vi "VI Tree.vi"   [LabVIEW 2012, in "Temptronic TP04300.lvlib"]
doc: "This is the instrument driver for the Temptronic 4300. The VI Tree displays all the user-callable VIs of the instrument driver in an organized table."
uses:
  <instrlib>/Temptronic TP04300/Temptronic TP04300.lvlib
panel:
  # "© 2007 Temptronic Corporation.  ALL RIGHTS RESERVED."
  # "SEE DIAGRAM\nFOR VI TREE."
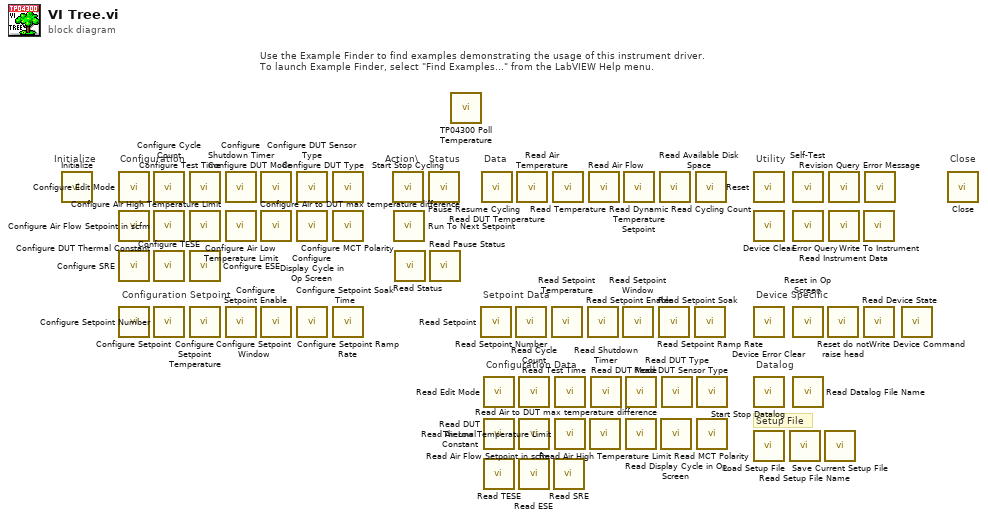
[diagram p0: block diagram]
diagram:
  # "Device Specific"
  # "Configuration Data"
  # "Configuration"
  # "Setpoint Data"
  # "Configuration Setpoint"
  # "Datalog"
  # "Status"
  # "Setup File"
  # "Use the Example Finder to find examples demonstrating the usage of this instrument driver.\nTo launch Example Finder, select \"Find Examples...\" from the LabVIEW Help menu."
  # "Utility"
  # "Data"
  # "Action\\"
  # "Close"
  # "Initialize"
  n1 = call <instrlib>:"Initialize.vi"() -> ()  [unwired: 10 in, 2 out]
  n2 = call <instrlib>:"Configure Edit Mode.vi"() -> ()  [unwired: 10 in, 2 out]
  n3 = call <instrlib>:"Configure DUT Thermal Constant.vi"() -> ()  [unwired: 10 in, 2 out]
  n4 = call <instrlib>:"Configure SRE.vi"() -> ()  [unwired: 10 in, 2 out]
  n5 = call <instrlib>:"Configure Setpoint.vi"() -> ()  [unwired: 10 in, 2 out]
  n6 = call <instrlib>:"Configure Cycle Count.vi"() -> ()  [unwired: 10 in, 2 out]
  n7 = call <instrlib>:"Configure Air Flow Setpoint in scfm.vi"() -> ()  [unwired: 10 in, 2 out]
  n8 = call <instrlib>:"Configure TESE.vi"() -> ()  [unwired: 10 in, 2 out]
  n9 = call <instrlib>:"Configure Setpoint Number.vi"() -> ()  [unwired: 10 in, 2 out]
  n10 = call <instrlib>:"Configure Test Time.vi"() -> ()  [unwired: 10 in, 2 out]
  n11 = call <instrlib>:"Configure Air High Temperature Limit.vi"() -> ()  [unwired: 10 in, 2 out]
  n12 = call <instrlib>:"Configure ESE.vi"() -> ()  [unwired: 10 in, 2 out]
  n13 = call <instrlib>:"Configure Setpoint Temperature.vi"() -> ()  [unwired: 10 in, 2 out]
  n14 = call <instrlib>:"Configure Shutdown Timer.vi"() -> ()  [unwired: 10 in, 2 out]
  n15 = call <instrlib>:"Configure Air Low Temperature Limit.vi"() -> ()  [unwired: 10 in, 2 out]
  n16 = call <instrlib>:"Configure Setpoint Enable.vi"() -> ()  [unwired: 10 in, 2 out]
  n17 = call <instrlib>:"Configure DUT Mode.vi"() -> ()  [unwired: 10 in, 2 out]
  n18 = call <instrlib>:"Configure Air to DUT max temperature difference.vi"() -> ()  [unwired: 10 in, 2 out]
  n19 = call <instrlib>:"Configure Setpoint Window.vi"() -> ()  [unwired: 10 in, 2 out]
  n20 = call <instrlib>:"Configure DUT Sensor Type.vi"() -> ()  [unwired: 10 in, 2 out]
  n21 = call <instrlib>:"Configure Display Cycle in Op Screen.vi"() -> ()  [unwired: 10 in, 2 out]
  n22 = call <instrlib>:"Configure Setpoint Soak Time.vi"() -> ()  [unwired: 10 in, 2 out]
  n23 = call <instrlib>:"Configure DUT Type.vi"() -> ()  [unwired: 10 in, 2 out]
  n24 = call <instrlib>:"Configure MCT Polarity.vi"() -> ()  [unwired: 10 in, 2 out]
  n25 = call <instrlib>:"Configure Setpoint Ramp Rate.vi"() -> ()  [unwired: 10 in, 2 out]
  n26 = call <instrlib>:"Start Stop Cycling.vi"() -> ()  [unwired: 10 in, 2 out]
  n27 = call <instrlib>:"Run To Next Setpoint.vi"() -> ()  [unwired: 10 in, 2 out]
  n28 = call <instrlib>:"Read Status.vi"() -> ()  [unwired: 9 in, 3 out]
  n29 = call <instrlib>:"Pause Resume Cycling.vi"() -> ()  [unwired: 10 in, 2 out]
  n30 = call <instrlib>:"Read Pause Status.vi"() -> ()  [unwired: 9 in, 3 out]
  n31 = call <instrlib>:"TP04300 Poll Temperature.vi"() -> ()  [unwired: 1 in]
  n32 = call <instrlib>:"Read Setpoint.vi"() -> ()  [unwired: 9 in, 3 out]
  n33 = call <instrlib>:"Read DUT Temperature.vi"() -> ()  [unwired: 9 in, 3 out]
  n34 = call <instrlib>:"Read Edit Mode.vi"() -> ()  [unwired: 9 in, 3 out]
  n35 = call <instrlib>:"Read DUT Thermal Constant.vi"() -> ()  [unwired: 9 in, 3 out]
  n36 = call <instrlib>:"Read TESE.vi"() -> ()  [unwired: 9 in, 3 out]
  n37 = call <instrlib>:"Read Setpoint Number.vi"() -> ()  [unwired: 9 in, 3 out]
  n38 = call <instrlib>:"Read Air Temperature.vi"() -> ()  [unwired: 9 in, 3 out]
  n39 = call <instrlib>:"Read Cycle Count.vi"() -> ()  [unwired: 9 in, 3 out]
  n40 = call <instrlib>:"Read Air Flow Setpoint in scfm.vi"() -> ()  [unwired: 9 in, 3 out]
  n41 = call <instrlib>:"Read ESE.vi"() -> ()  [unwired: 9 in, 3 out]
  n42 = call <instrlib>:"Read Setpoint Temperature.vi"() -> ()  [unwired: 9 in, 3 out]
  n43 = call <instrlib>:"Read Temperature.vi"() -> ()  [unwired: 9 in, 3 out]
  n44 = call <instrlib>:"Read SRE.vi"() -> ()  [unwired: 9 in, 3 out]
  n45 = call <instrlib>:"Read Test Time.vi"() -> ()  [unwired: 9 in, 3 out]
  n46 = call <instrlib>:"Read Air Low Temperature Limit.vi"() -> ()  [unwired: 9 in, 3 out]
  n47 = call <instrlib>:"Read Setpoint Enable.vi"() -> ()  [unwired: 9 in, 3 out]
  n48 = call <instrlib>:"Read Air Flow.vi"() -> ()  [unwired: 8 in, 4 out]
  n49 = call <instrlib>:"Read Air High Temperature Limit.vi"() -> ()  [unwired: 9 in, 3 out]
  n50 = call <instrlib>:"Read Shutdown Timer.vi"() -> ()  [unwired: 9 in, 3 out]
  n51 = call <instrlib>:"Read Setpoint Window.vi"() -> ()  [unwired: 9 in, 3 out]
  n52 = call <instrlib>:"Read Dynamic Temperature Setpoint.vi"() -> ()  [unwired: 9 in, 3 out]
  n53 = call <instrlib>:"Read DUT Mode.vi"() -> ()  [unwired: 9 in, 3 out]
  n54 = call <instrlib>:"Read Air to DUT max temperature difference.vi"() -> ()  [unwired: 9 in, 3 out]
  n55 = call <instrlib>:"Read Setpoint Soak.vi"() -> ()  [unwired: 9 in, 3 out]
  n56 = call <instrlib>:"Read Available Disk Space.vi"() -> ()  [unwired: 9 in, 3 out]
  n57 = call <instrlib>:"Read Display Cycle in Op Screen.vi"() -> ()  [unwired: 9 in, 3 out]
  n58 = call <instrlib>:"Read DUT Type.vi"() -> ()  [unwired: 9 in, 3 out]
  n59 = call <instrlib>:"Read Setpoint Ramp Rate.vi"() -> ()  [unwired: 9 in, 3 out]
  n60 = call <instrlib>:"Read Cycling Count.vi"() -> ()  [unwired: 9 in, 3 out]
  n61 = call <instrlib>:"Read DUT Sensor Type.vi"() -> ()  [unwired: 9 in, 3 out]
  n62 = call <instrlib>:"Read MCT Polarity.vi"() -> ()  [unwired: 9 in, 3 out]
  n63 = call <instrlib>:"Reset.vi"() -> ()  [unwired: 10 in, 2 out]
  n64 = call <instrlib>:"Device Clear.vi"() -> ()  [unwired: 10 in, 2 out]
  n65 = call <instrlib>:"Device Error Clear.vi"() -> ()  [unwired: 10 in, 2 out]
  n66 = call <instrlib>:"Start Stop Datalog.vi"() -> ()  [unwired: 10 in, 2 out]
  n67 = call <instrlib>:"Load Setup File.vi"() -> ()  [unwired: 10 in, 2 out]
  n68 = call <instrlib>:"Read Setup File Name.vi"() -> ()  [unwired: 9 in, 3 out]
  n69 = call <instrlib>:"Self-Test.vi"() -> ()  [unwired: 8 in, 4 out]
  n70 = call <instrlib>:"Error Query.vi"() -> ()  [unwired: 8 in, 4 out]
  n71 = call <instrlib>:"Reset in Op Screen.vi"() -> ()  [unwired: 10 in, 2 out]
  n72 = call <instrlib>:"Read Datalog File Name.vi"() -> ()  [unwired: 9 in, 3 out]
  n73 = call <instrlib>:"Save Current Setup File.vi"() -> ()  [unwired: 10 in, 2 out]
  n74 = call <instrlib>:"Reset do not raise head.vi"() -> ()  [unwired: 10 in, 2 out]
  n75 = call <instrlib>:"Revision Query.vi"() -> ()  [unwired: 8 in, 4 out]
  n76 = call <instrlib>:"Read Instrument Data.vi"() -> ()  [unwired: 8 in, 4 out]
  n77 = call <instrlib>:"Write To Instrument.vi"() -> ()  [unwired: 10 in, 2 out]
  n78 = call <instrlib>:"Read Device State.vi"() -> ()  [unwired: 8 in, 4 out]
  n79 = call <instrlib>:"Error Message.vi"() -> ()  [unwired: 9 in, 3 out]
  n80 = call <instrlib>:"Write Device Command.vi"() -> ()  [unwired: 10 in, 2 out]
  n81 = call <instrlib>:"Close.vi"() -> ()  [unwired: 11 in, 1 out]
